vi "memory to strings.vi"(8 "error in":errorcluster, 11 "memory hierarchy":T5) -> (0 "error out":errorcluster, 3 "1.0.0":T1)   [LabVIEW 2025, in "CEF.lvlib"]
doc: "Flattens an object hierarchy into a flattened instance set version 1.0.0.Copyright 2017 National Instruments Corporation\n\nLicensed under the Apache License, Version 2.0 (the \"License\"); you may not use this file except in compliance with the License. You may obtain a copy of the License at http://www.apache.org/licenses/LICENSE-2.0\nUnless required by applicable law or agreed to in writing, software distributed under the License is distributed on an \"AS IS\" BASIS, WITHOUT WARRANTIES OR CONDITIONS OF ANY KIND, either express or implied. See the License for the specific language governing permissions and limitations under the License."
uses:
  CEF.lvlib
  hierarchy repo/memory hierarchy.ctl
  hierarchy repo/full hierarchy.ctl
  hierarchy element.ctl
  serializable configuration/CEF_serializable configuration.lvclass
  flat hierarchy.ctl
  instance data.ctl
  serializable configuration/CEF_serializable configuration.lvclass/CEF_serializable configuration.ctl
  <vilib>/Utility/LVClass/Get LV Class Name.vi
  error generator/CEF_error generator.vi
  hierarchy repo/CEF_HierarchyRepo.lvclass
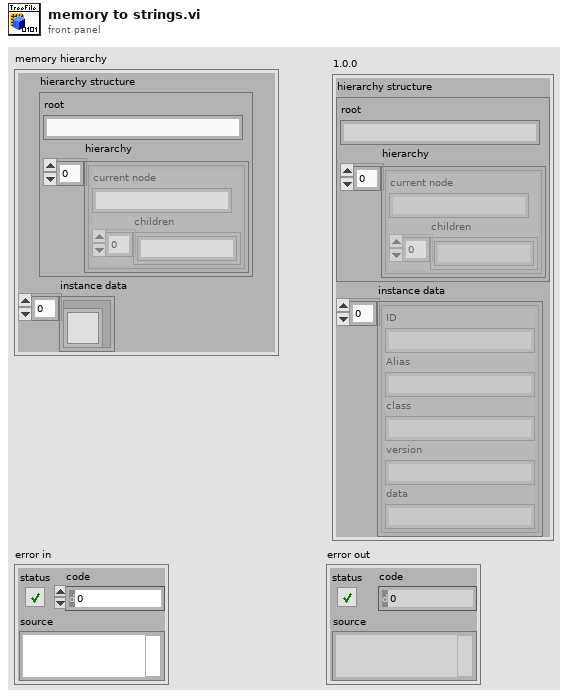
[diagram p1: front panel]
types:
  T1 = typedef "CEF.lvlib/flat hierarchy.ctl" = cluster{"hierarchy structure":T2, "instance data":T4[]}
  T2 = typedef "CEF.lvlib/CEF_HierarchyRepo.lvclass/full hierarchy.ctl" = cluster{"root":string, "hierarchy":T3[]}
  T3 = typedef "CEF.lvlib/hierarchy element.ctl" = cluster{"current node":string, "children":string[]}
  T4 = typedef "CEF.lvlib/instance data.ctl" = cluster{"ID":string, "Alias":string, "class":string, "version":string, "data":string}
  T5 = typedef "CEF.lvlib/CEF_HierarchyRepo.lvclass/memory hierarchy.ctl" = cluster{"hierarchy structure":T2, "instance data":refnum<class "CEF_serializable configuration.lvclass">[]}
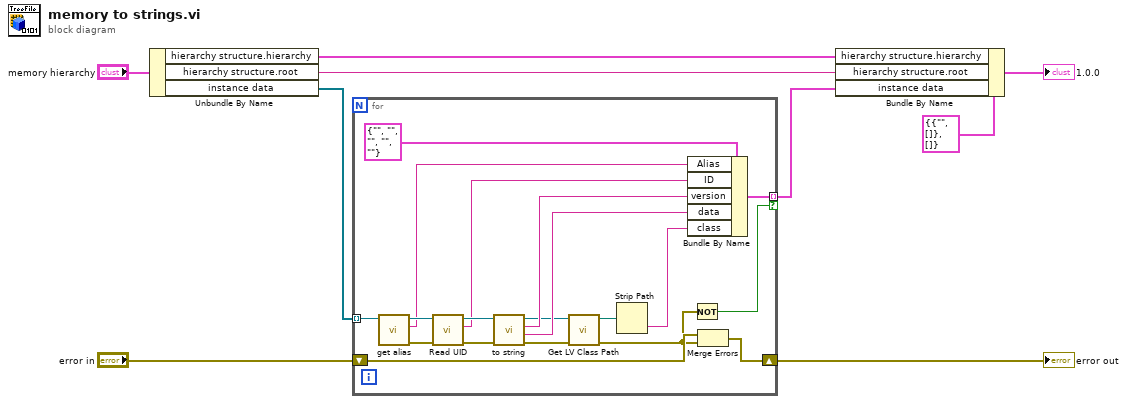
[diagram p0: block diagram]
diagram:
  n1 = Unbundle By Name("memory hierarchy") -> ("hierarchy structure.hierarchy"=w4:T3[], "hierarchy structure.root"=w3:string, "instance data"=w2:refnum<class "CEF_serializable configuration.lvclass">[])
  n2 = for {
    tunnel: [w27] -> w1 mode=indexing if=w14
    tunnel: w2 -> [w20] mode=indexing
    shift-right: [w21] -> w7
    shift-left: "error in" -> [w22]
    n3 = call "get alias.vi"("CEF_Configuration in"=w20) -> ("error out"=w23:errorcluster, "alias"=w17:string, "CEF_Configuration out"=w19:refnum<class "CEF_serializable configuration.lvclass">)  [unwired: 8 in]
    n4 = call "Read UID.vi"("error in"=w23, "CEF_Configuration in"=w19) -> ("error out"=w16:errorcluster, "instance id"=w18:string, "CEF_Configuration out"=w24:refnum<class "CEF_serializable configuration.lvclass">)  [unwired: 7 in]
    n5 = call-dynamic "to string.vi"("error in"=w16, "CEF_Configuration in"=w24) -> ("error out"=w15:errorcluster, "data"=w13:string, "version"=w25:string, "CEF_Configuration out"=w10:refnum<class "CEF_serializable configuration.lvclass">)  [unwired: 6 in]
    n6 = call <vilib>:"Get LV Class Path.vi"("error in (no error)"=w15, "object"=w10) -> ("error out"=w11:errorcluster, "class path"=w26:path)  [unwired: 8 in]
    n7 = Strip Path(path=w26) -> (name=w12:string)  [unwired: 1 out]
    n8 = Bundle By Name(cluster=T4 {"ID"="", "Alias"="", "class"="", "version"="", "data"=""} ("instancedata"), "Alias"=w17, "ID"=w18, "version"=w25, "data"=w13, "class"=w12) -> (w27:T4)
    n9 = Not(x=w11) -> (.not. x?=w14:bool)
    n10 = Merge Errors(w22, w11) -> (w21:errorcluster)
  }
  "error out" <- w7
  n11 = Bundle By Name(cluster=T1 {"hierarchy structure"={"root"="", "hierarchy"=[]}, "instance data"=[]} ("1.0.0"), "hierarchy structure.hierarchy"=w4, "hierarchy structure.root"=w3, "instance data"=w1) -> (→"1.0.0":T1)
